vi "Poly Set Map Verify New Type.vi"(5 "Poly Set Map":T2, 7 "Poly Ref Map":T1, 9 "Selector Name":string, 10 "Menu Name":string, 11 "Directory":path) -> (2 "Valid?":bool, 3 "Error Message":string)   [LabVIEW 2020]
uses:
  _td_map_PolyInstanceInfo.ctl
  _td_cluster_InstanceInfo.ctl
  _td_map_PolyRef.ctl
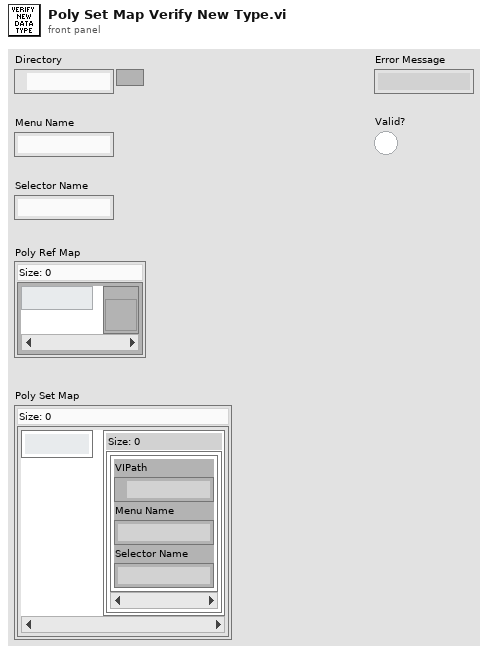
[diagram p1: front panel]
types:
  T1 = typedef "_td_map_PolyRef.ctl" = map{string, refnum<vi>}
  T2 = typedef "_td_map_PolyInstanceInfo.ctl" = map{string, set{T3}}
  T3 = typedef "_td_cluster_InstanceInfo.ctl" = cluster{"VIPath":path, "Menu Name":string, "Selector Name":string}
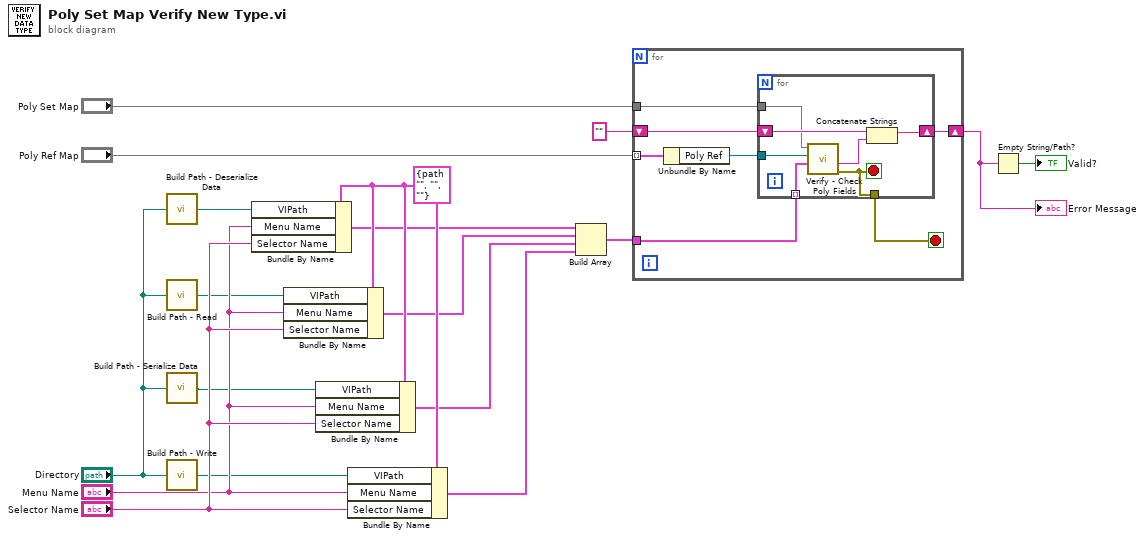
[diagram p0: block diagram]
diagram:
  w15 = T3 {"VIPath"=path "", "Menu Name"="", "Selector Name"=""} ("InstanceInfo")
  n1 = call "Build Path - Deserialize Data.vi"("Directory"="Directory") -> ("Path to Deserialize Data.vi"=w16:path)
  n2 = call "Build Path - Read.vi"("Directory"="Directory") -> ("Path to Read.vi"=w3:path)
  n3 = call "Build Path - Serialize Data.vi"("Directory"="Directory") -> ("Path to Serialize Data.vi"=w4:path)
  n4 = call "Build Path - Write.vi"("Directory"="Directory") -> ("Path to Write.vi"=w5:path)
  n5 = Bundle By Name(cluster=w15, "VIPath"=w16, "Menu Name"="Menu Name", "Selector Name"="Selector Name") -> (w13:T3)
  n6 = Bundle By Name(cluster=w15, "VIPath"=w3, "Menu Name"="Menu Name", "Selector Name"="Selector Name") -> (w12:T3)
  n7 = Bundle By Name(cluster=w15, "VIPath"=w4, "Menu Name"="Menu Name", "Selector Name"="Selector Name") -> (w11:T3)
  n8 = Bundle By Name(cluster=w15, "VIPath"=w5, "Menu Name"="Menu Name", "Selector Name"="Selector Name") -> (w10:T3)
  n9 = Build Array(w13, w12, w11, w10) -> (w8:T3[])
  n10 = for {
    tunnel: "Poly Ref Map" -> [w25] mode=indexing
    tunnel: w8 -> [w23]
    shift-right: [w22] -> w6
    shift-left: "" ("Error?") -> [w21]
    tunnel: "Poly Set Map" -> [w19]
    stop <- w20 stop-if-true
    n11 = Unbundle By Name(w25) -> ("Poly Ref"=w24:refnum<vi>)
    n12 = for {
      tunnel: w24 -> [w32]
      tunnel: w23 -> [w31] mode=indexing
      shift-right: [w28] -> w22
      shift-left: w21 -> [w29]
      tunnel: [w27] -> w20
      tunnel: w19 -> [w26]
      stop <- w27 stop-if-true
      n13 = call "Verify - Check Poly Fields.vi"("InstanceInfo"=w31, "Poly Ref"=w32, "Poly Map Set in"=w26) -> ("error out"=w27:errorcluster, "Error?"=w30:string)  [unwired: 7 in]
      n14 = Concatenate Strings(w29, w30) -> (w28:string)
    }
  }
  "Error Message" <- w6
  n15 = Empty String/Path?(string/path=w6) -> (empty?=→"Valid?":bool)
